vi "User2MotorTorque.vi"(11 "User Torque [Nm]":dbl) -> (3 "Motor Torque [Nm]":dbl)   [LabVIEW 2019]
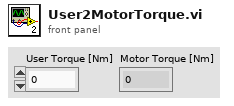
[diagram p1: front panel]
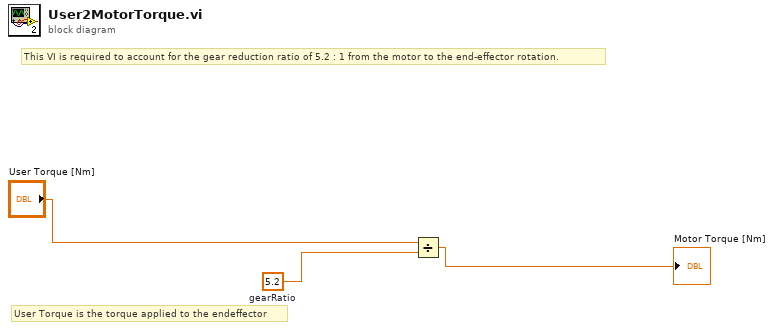
[diagram p0: block diagram]
diagram:
  w2 = 5.2  # gearRatio
  # "This VI is required to account for the gear reduction ratio of 5.2 : 1 from the motor to the end-effector rotation."
  # "User Torque is the torque applied to the endeffector"
  n1 = Divide(x="User Torque [Nm]", y=w2) -> (x/y=→"Motor Torque [Nm]":dbl)
